vi "Drop.vi"(11 "Response Core in":refnum<class "Interruptible Reply Core.lvclass">) -> ()   [LabVIEW 2020, in "Publisher.lvlib" / "Interruptible Reply Core.lvclass"]
doc: "Drop the Response Core.\n\nRelease the Reply Queue and the Interrupt Notifier. Force destroy on the Reply Queue."
uses:
  Interruptible Reply Core.lvclass
  Interruptible Reply Core.lvclass/Interruptible Reply Core.ctl
  PPL/HDH.Data.Generic.lvlibp/Synchronization/Queue/Queue.lvclass
  PPL/HDH.Data.Generic.lvlibp/Synchronization/Notifier/Notifier.lvclass
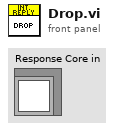
[diagram p1: front panel]
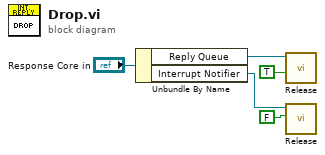
[diagram p0: block diagram]
diagram:
  n1 = Unbundle By Name("Response Core in") -> ("Reply Queue"=w4:refnum<class "Queue.lvclass">, "Interrupt Notifier"=w2:refnum<class "Notifier.lvclass">)
  n2 = call "Release.vi"("force destroy? (F)"=TRUE, "Queue in"=w4) -> ()  [unwired: 7 in, 3 out]
  n3 = call "Release.vi"("Force destroy? (F)"=FALSE, "Notifier in"=w2) -> ()  [unwired: 7 in, 3 out]
